vi "ID_step.vi"(11 "Sensor Readings":dbl[][][](array[numeric])) -> (1 "Start Index":i32, 2 "End Index":i32, 3 "Load Profile":dbl[](array[numeric]))   [LabVIEW 2018]
uses:
  <vilib>/Analysis/baseanly.llb/Mean (DBL).vi
  <vilib>/Analysis/NI_AALBase.lvlib
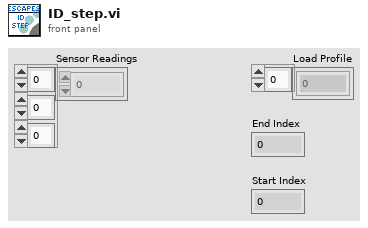
[diagram p1: front panel]
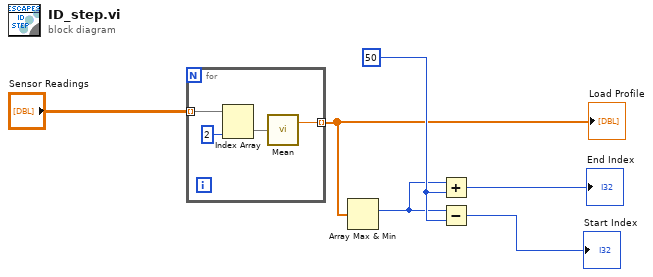
[diagram p0: block diagram]
diagram:
  w4 = 50 ("disabled index (col)")
  n1 = for {
    tunnel: "Sensor Readings" -> [w10] mode=indexing
    tunnel: [w7] -> w2 mode=indexing
    n2 = Index Array(array=w10, index (col)=2 ("disabled index (col)")) -> (element=w8:dbl[])  [unwired: 1 in]
    n3 = call-poly <vilib>:"Mean.vi"("X"=w8) -> ("mean"=w7:dbl)  [unwired: 1 out]
  }
  "Load Profile" <- w2
  n4 = Array Max & Min(array=w2) -> (max index (indices)=w3:i32)  [unwired: 3 out]
  n5 = Add(x=w3, y=w4) -> (x+y=→"End Index":i32)
  n6 = Subtract(x=w3, y=w4) -> (x-y=→"Start Index":i32)
